vi "Configure Module.vi"(8 "error in (no error)":errorcluster, 10 "IOV ref in":refnum<k21>, 11 "9235 in":refnum<class "9235.lvclass">) -> (0 "error out":errorcluster, 2 "IOV ref out":refnum<k21>, 3 "9235 out":refnum<class "9235.lvclass">)   [LabVIEW 2011, in "Modules.lvlib" / "9235.lvclass"]
uses:
  9235.lvclass
  9235.lvclass/9235.ctl
  Program Files (x86)/National Instruments/LabVIEW 2011/resource/objmgr/cRIO.rc
  RSI Module/RSI Module.lvclass
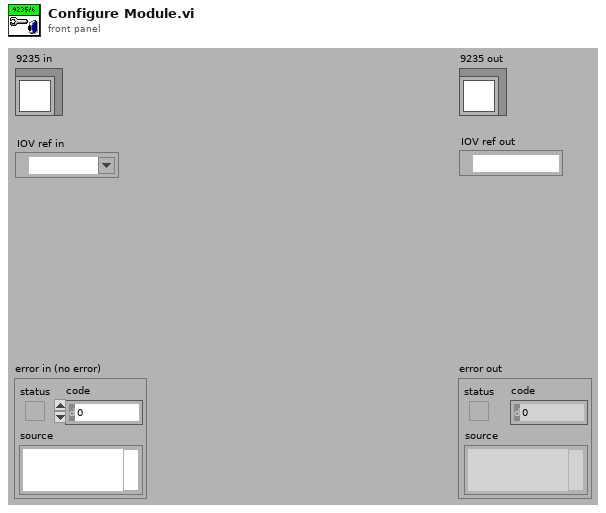
[diagram p1: front panel]
types:
  T1 = typedef "Modules.lvlib/RSI Module.lvclass/Module Models.ctl" = enum16{"Empty", "NI 9201", "NI 9203", "NI 9205", "NI 9206", "NI 9207", "NI 9208", "NI 9211", "NI 9213", "NI 9214", "NI 9215", "NI 9217", "NI 9219", "NI 9221", "NI 9225", "NI 9227", "NI 9229", "NI 9233", "NI 9234", "NI 9235", "NI 9236", "NI 9237", "NI 9239", "NI 9263", "NI 9264", "NI 9265", "NI 9269", "NI 9375", "NI 9401", "NI 9402", "NI 9403", "NI 9411", "NI 9421", "NI 9422", "NI 9423", "NI 9425", "NI 9426", "NI 9435", "NI 9472", "NI 9474", "NI 9475", "NI 9476", "NI 9477", "NI 9478", "NI 9481", "NI 9482", "NI 9485"}
  T2 = typedef "Modules.lvlib/9235.lvclass/Data rate.ctl" = u32
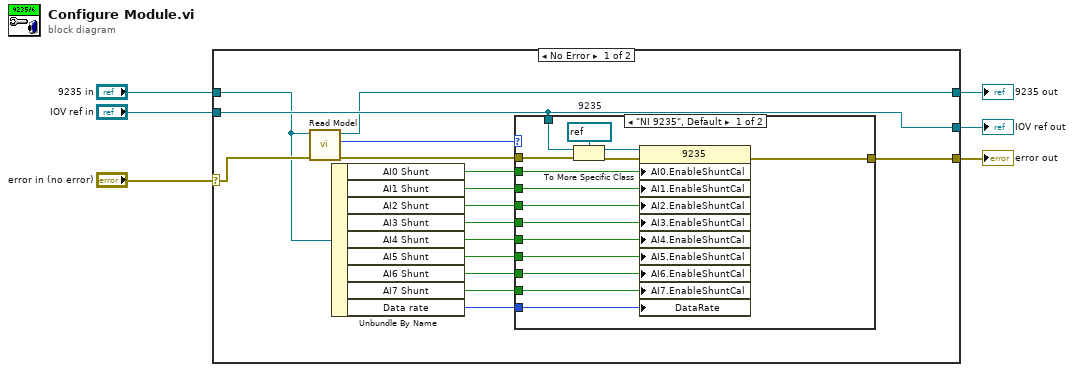
[diagram p0: block diagram]
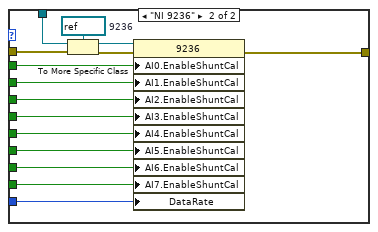
[diagram p2: hidden frame]
diagram:
  n1 = case shown="No Error" "error in (no error)" {
    selector: "error in (no error)" -> [w11 w55]
    tunnel: [w12 w55] -> w5
    tunnel: [w8 w54] -> w3
    tunnel: "9235 in" -> [w9 w54]
    tunnel: "IOV ref in" -> [w22 w53]
    tunnel: [w22 w53] -> w1
    frame No Error {
      n2 = call "Read Model.vi"("error in (no error)"=w11, "RSI Module in"=w9) -> ("error out"=w10:errorcluster, "Model"=w7:T1, "RSI Module out"=w8:refnum<class "9235.lvclass">)  [unwired: 7 in]
      n3 = Unbundle By Name(w9) -> ("AI0 Shunt"=w21:bool, "AI1 Shunt"=w20:bool, "AI2 Shunt"=w19:bool, "AI3 Shunt"=w18:bool, "AI4 Shunt"=w17:bool, "AI5 Shunt"=w16:bool, "AI6 Shunt"=w15:bool, "AI7 Shunt"=w14:bool, "Data rate"=w13:T2)
      n4 = case shown="\"NI 9235\", Default" w7 {
        tunnel: w22 -> [w35 w50]
        tunnel: w21 -> [w33 w48]
        tunnel: w20 -> [w32 w47]
        tunnel: w19 -> [w31 w46]
        tunnel: w18 -> [w30 w45]
        tunnel: w17 -> [w29 w44]
        tunnel: w16 -> [w28 w43]
        tunnel: w15 -> [w27 w42]
        tunnel: w14 -> [w26 w41]
        tunnel: w13 -> [w25 w40]
        tunnel: [w24 w39] -> w12
        tunnel: w10 -> [w23 w38]
        frame "NI 9235", Default {
          w37 = refnum<k21> refnum  # 9235
          n5 = To More Specific Class(target class=w37, reference=w35, error in=w23) -> (specific class reference=w34:refnum<k21>, error out=w36:errorcluster)
          n6 = property class="9235"(reference=w34, error in=w36, "AI0.EnableShuntCal"=w33, "AI1.EnableShuntCal"=w32, "AI2.EnableShuntCal"=w31, "AI3.EnableShuntCal"=w30, "AI4.EnableShuntCal"=w29, "AI5.EnableShuntCal"=w28, "AI6.EnableShuntCal"=w27, "AI7.EnableShuntCal"=w26, "DataRate"=w25) -> (error out=w24:errorcluster)  [unwired: 1 out]
        }
        frame "NI 9236" {
          w52 = refnum<k21> refnum  # 9236
          n7 = To More Specific Class(target class=w52, reference=w50, error in=w38) -> (specific class reference=w49:refnum<k21>, error out=w51:errorcluster)
          n8 = property class="9236"(reference=w49, error in=w51, "AI0.EnableShuntCal"=w48, "AI1.EnableShuntCal"=w47, "AI2.EnableShuntCal"=w46, "AI3.EnableShuntCal"=w45, "AI4.EnableShuntCal"=w44, "AI5.EnableShuntCal"=w43, "AI6.EnableShuntCal"=w42, "AI7.EnableShuntCal"=w41, "DataRate"=w40) -> (error out=w39:errorcluster)  [unwired: 1 out]
        }
      }
    }
    frame Error {
    }
  }
  "error out" <- w5
  "9235 out" <- w3
  "IOV ref out" <- w1
